vi "Find Sparks by Step Detection.vi"(3 "error in (no error)":errorcluster, 4 "Min Spark Length":i32=5000, 5 "Waveform":dbl[](array[numeric])) -> (0 "error out":errorcluster, 2 "Spark Indicies":i32[](array[numeric]))   [LabVIEW 2012]
panel:
  out "Converged":bool
  out "Waveform Graph":dbl[][](graph)
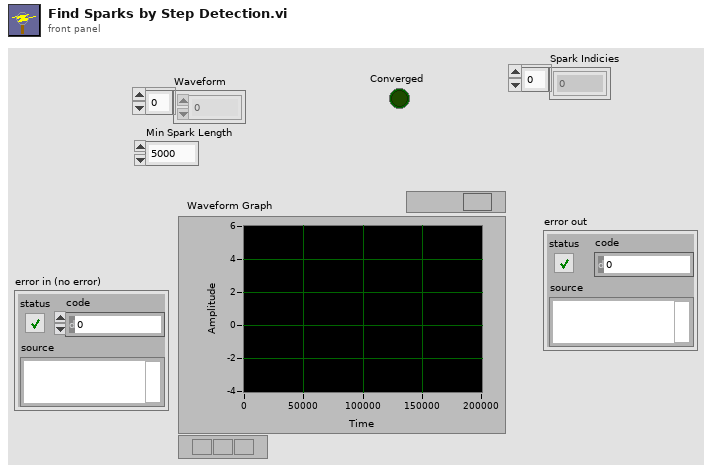
[diagram p1: front panel]
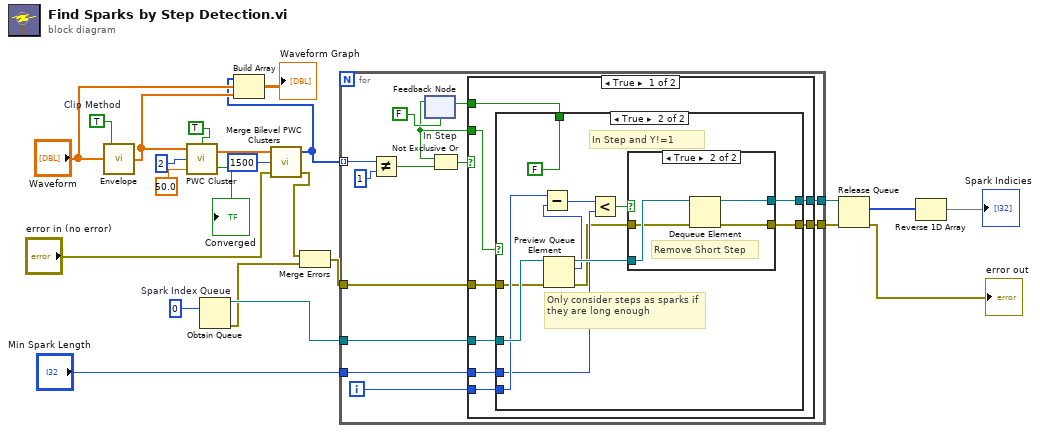
[diagram p0: block diagram]
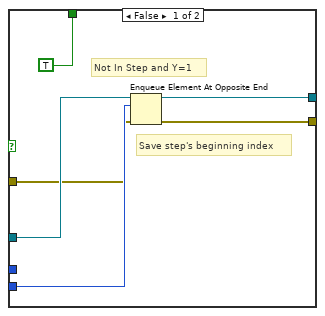
[diagram p2: hidden frame]
diagram:
  w1 = TRUE  # Clip Method
  n1 = call "Envelope.vi"("Waveform"="Waveform", "Hilbert Transform/Clip Method"=w1) -> ("Envelope"=w7:dbl[])  [unwired: 3 in]
  n2 = call "PWC Cluster.vi"("Return Indicies"=TRUE, "Kernel Precission Parameter"=50.0 ("Kernel Parameter/Support"), "# Cluster Levels"=2, "Input Waveform"=w7) -> ("Converged"=→"Converged":bool, "Cluster Assignments"=w6:dbl[])
  n3 = Obtain Queue "Spark Index Queue"(element data type=0 ("# Cluster Levels")) -> (queue out=w22:refnum<queue>, error out=w12:errorcluster)  [unwired: 4 in, 1 out]
  n4 = call "Merge Bilevel PWC Clusters.vi"("error in (no error)"="error in (no error)", "Max Gap Length"=1500, "Bilevel PWC Waveform"=w6) -> ("error out"=w2:errorcluster, "Merged Bilevel PWC Waveform"=w3:i32[])  [unwired: 1 in]
  n5 = Build Array(w3, "Waveform", w7) -> (→"Waveform Graph":dbl[][])
  n6 = Merge Errors(w2, w12) -> (w11:errorcluster)
  n7 = for {
    tunnel: w3 -> [w26] mode=indexing
    tunnel: w22 -> [w33]
    tunnel: [w32] -> w20
    tunnel: "Min Spark Length" -> [w31]
    tunnel: w11 -> [w25]
    tunnel: [w24] -> w10
    i -> [w27]
    n8 = Not Equal?(x=w26, y=1) -> (x != y?=w30:bool)
    n9 = feedback #1 "In Step"(FALSE) -> (w29:bool)
    n10 = Not Exclusive Or(1:w30, 2:w29) -> (0:w28:bool)
    n11 = case shown="True" w28 {
      tunnel: [w40 w70] -> w34
      tunnel: w33 -> [w44 w71]
      tunnel: [w43 w71] -> w32
      tunnel: w29 -> [w41 w70]
      tunnel: w31 -> [w39 _]
      tunnel: w27 -> [w42 _]
      tunnel: w25 -> [w38 w69]
      tunnel: [w37 w69] -> w24
      frame True {
        n12 = case shown="True" w41 {
          tunnel: w44 -> [w50 w56]
          tunnel: [w49 w57] -> w43
          tunnel: w42 -> [w48 w55]
          tunnel: [TRUE FALSE] -> w40
          tunnel: w39 -> [_ w54]
          tunnel: w38 -> [w46 w53]
          tunnel: [w45 w51] -> w37
          frame False {
            # "Save step's beginning index"
            # "Not In Step and Y=1"
            n13 = Enqueue Element At Opposite End(queue=w50, element=w48, error in (no error)=w46) -> (queue out=w49:refnum<queue>, error out=w45:errorcluster)  [unwired: 1 in, 1 out]
          }
          frame True {
            # "Only consider steps as sparks if they are long enough"
            # "In Step and Y!=1"
            n14 = Preview Queue Element(queue=w56, error in (no error)=w53) -> (queue out=w60:refnum<queue>, element=w59:i32, error out=w52:errorcluster)  [unwired: 1 in, 1 out]
            n15 = Subtract(x=w55, y=w59) -> (x-y=w58:i32)
            n16 = Less?(x=w58, y=w54) -> (x < y?=w61:bool)
            n17 = case shown="True" w61 {
              tunnel: w60 -> [w64 w68]
              tunnel: [w64 w67] -> w57
              tunnel: w52 -> [w63 w66]
              tunnel: [w63 w65] -> w51
              frame False {
                # "Keep Long Step (Spark)"
              }
              frame True {
                # "Remove Short Step"
                n18 = Dequeue Element(queue=w68, error in (no error)=w66) -> (queue out=w67:refnum<queue>, error out=w65:errorcluster)  [unwired: 1 in, 2 out]
              }
            }
          }
        }
      }
      frame False {
      }
    }
    n19 = feedback-in #1(w34) -> ()
  }
  n20 = Release Queue(queue=w20, error in (no error)=w10) -> (remaining elements=w16:i32[], error out=→"error out":errorcluster)  [unwired: 1 in, 1 out]
  n21 = Reverse 1D Array(array=w16) -> (reversed array=→"Spark Indicies":i32[])
